vi "Open or Create Event Log File.vi"(11 "Filename In":string) -> (0 "error out":errorcluster, 3 "refnum out":refnum<file>)   [LabVIEW 2020]
doc: "The \"Open or Create Event Log File\" subVI takes as input the name for the event log text file. It then builds an application directory in the same relative location as the main VI. Then it checks if the file exists. If it does not, it creates a new file and writes a header to it. If the file does exist, it opens the file and appends all written event logs to the end of the file. This subVI then outputs the event log file refnum and error cluster."
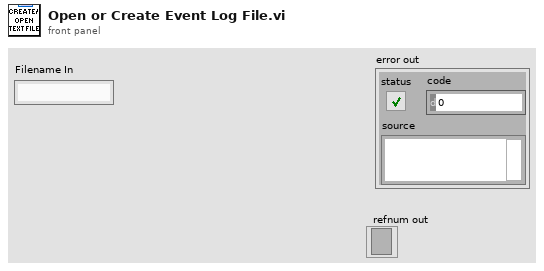
[diagram p1: front panel]
types:
  T1 = enum16{"open", "replace", "create", "open or create", "replace or create", "replace or create with confirmation"}
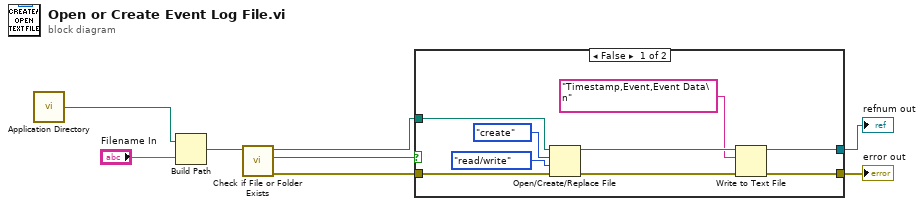
[diagram p0: block diagram]
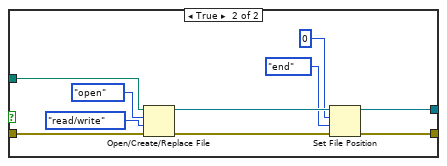
[diagram p2: hidden frame]
diagram:
  n1 = call <vilib>:"Application Directory.vi"() -> ("Application Directory"=w3:path)
  n2 = Build Path(base path=w3, name or relative path="Filename In") -> (appended path=w2:path)
  n3 = call <vilib>:"Check if File or Folder Exists.vi"("path"=w2) -> ("error out"=w6:errorcluster, "file or folder exists?"=w8:bool, "dup path"=w7:path)  [unwired: 8 in]
  n4 = case shown="False" w8 {
    tunnel: w7 -> [w17 w25]
    tunnel: w6 -> [w16 w24]
    tunnel: [w10 w20] -> w5
    tunnel: [w11 w21] -> w4
    frame False {
      n5 = Open/Create/Replace File(file path (use dialog)=w17, error in=w16, operation (0:open)=T1."create", access (0:read/write)=enum16{"read/write", "read-only", "write-only"}."read/write") -> (refnum out=w13:refnum<file>, error out=w12:errorcluster)  [unwired: 2 in, 1 out]
      n6 = Write to Text File(file (use dialog)=w13, text="Timestamp,Event,Event Data\n", error in=w12) -> (refnum out=w11:refnum<file>, error out=w10:errorcluster)  [unwired: 1 in, 1 out]
    }
    frame True {
      n7 = Open/Create/Replace File(file path (use dialog)=w25, error in=w24, operation (0:open)=T1."open", access (0:read/write)=enum16{"read/write", "read-only", "write-only"}."read/write") -> (refnum out=w23:refnum<file>, error out=w22:errorcluster)  [unwired: 2 in, 1 out]
      n8 = Set File Position(offset (in bytes) (0)=i64 0, refnum=w23, from (0:start)=enum16{"start", "end", "current"}."end", error in=w22) -> (refnum out=w21:refnum<file>, error out=w20:errorcluster)
    }
  }
  "error out" <- w5
  "refnum out" <- w4
